vi "Move Sort Label.vi"(8 "error in (no error)":errorcluster, 10 "Target Label":refnum<vi>, 11 "Sort":refnum<vi>) -> (0 "error out":errorcluster)   [LabVIEW 2020, in "UI Common.lvlib"]
uses:
  UI Common.lvlib
  Sort Button.ctl
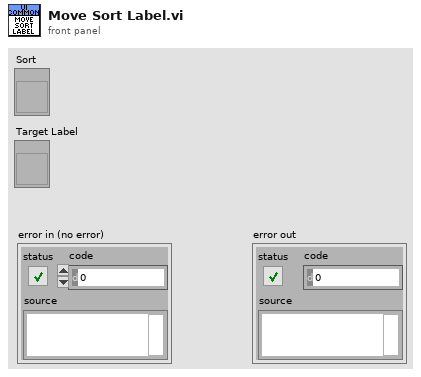
[diagram p1: front panel]
types:
  T1 = typedef "LVPositionTypeDef.ctl" = cluster{"Left":i32, "Top":i32}
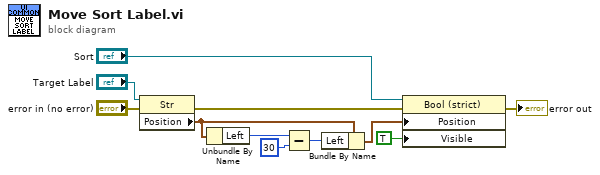
[diagram p0: block diagram]
diagram:
  n1 = property class="Str"(reference="Target Label", error in="error in (no error)") -> (error out=w9:errorcluster, "Position"=w7:T1)  [unwired: 1 out]
  n2 = Unbundle By Name(w7) -> ("Left"=w4:i32)
  n3 = Subtract(x=w4, y=30) -> (x-y=w6:i32)
  n4 = Bundle By Name(cluster=w7, "Left"=w6) -> (w8:T1)
  n5 = property class="Bool (strict)"(reference="Sort", error in=w9, "Position"=w8, "Visible"=TRUE) -> (error out=→"error out":errorcluster)  [unwired: 1 out]
